vi "KeyUp.vi"(2 "error in (no error)":errorcluster, 3 "Virtual Key":u8(ring)=65) -> (0 "error out":errorcluster)   [LabVIEW 2013]
uses:
  user32.dll
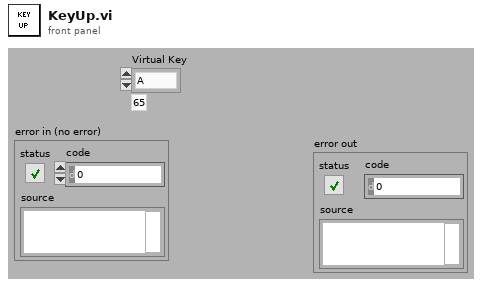
[diagram p1: front panel]
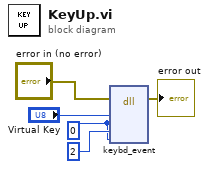
[diagram p0: block diagram]
diagram:
  w4 = u8 0 ("bScan")
  n1 = dll-call lib="user32.dll" fn="keybd_event"(error in="error in (no error)", "bVk"="Virtual Key", "bScan"=w4, "dwFlags"=u32 2, "dwExtraInfo"=w4) -> (error out=→"error out":errorcluster)  [unwired: 7 in, 1 out]
